vi "Stimulus-Set Level.vi"(0 "Level":T1, 1 "Apply multiplier? (F)":bool, 2 "Name":string, 5 "Waveform in":dbl[](array[numeric]), 11 "error in (no error)":errorcluster) -> (4 "Level out":T1, 6 "Waveform out":dbl[](array[numeric]), 8 "Multiplier":dbl, 10 "Ceiling":dbl, 15 "error out":errorcluster)   [LabVIEW 2020]
uses:
  Controls/Level XCtl/Level Data.ctl
  Controls/Level XCtl/Level Units.ctl
  PXI DAQ VIs/DAQ Engine VIs/PXI Globals.vi
  Utility VIs/Math VIs/dB to Linear (scalar).vi
  Controls/Level XCtl/Level XCtl.xctl
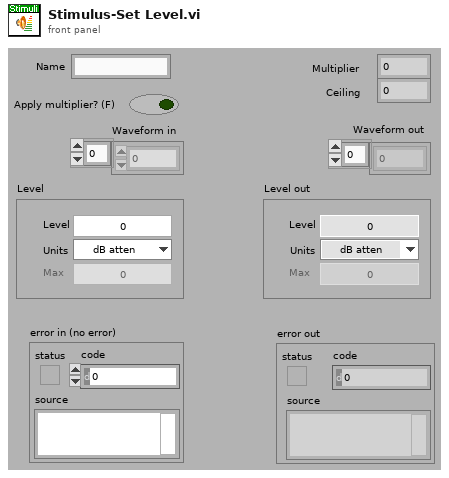
[diagram p1: front panel]
types:
  T1 = typedef "Level XCtl.xctl/Level Data.ctl" = cluster{"Level":dbl, "Units":T2, "Max":dbl, "Multiplier":dbl, "Cal File":path, "Cal":cluster{"Freq (Hz)":dbl[], "Mag (dB SPL)":dbl[], "Phase (deg)":dbl[]}}
  T2 = typedef "Level Units.ctl" = enum16{"dB atten", "dB SPL", "dB re 1 Vrms", "dB V/Hz½", "mW", "dB HL", "Volts", "dB mW"}
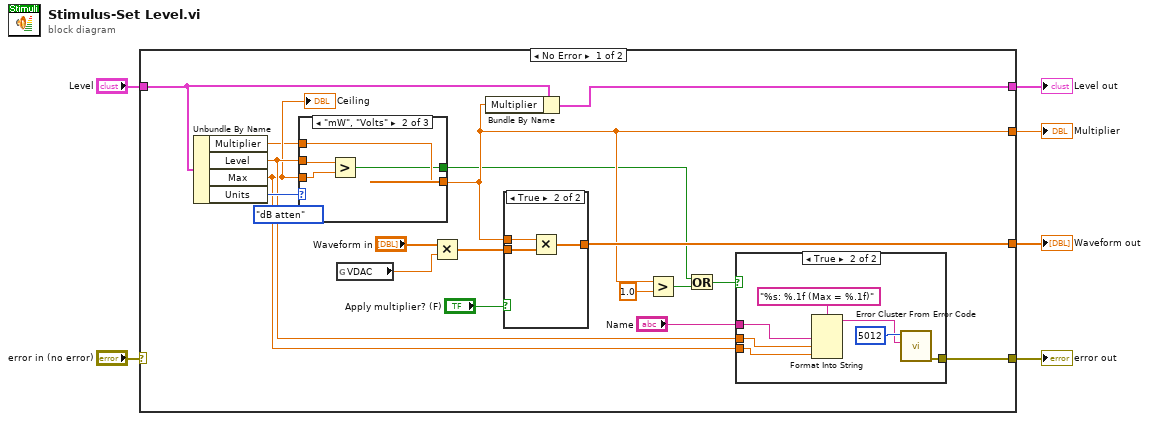
[diagram p0: block diagram]
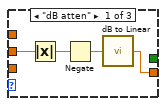
[diagram p4: hidden frame]
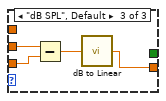
[diagram p5: hidden frame]
diagram:
  n1 = case shown="No Error" "error in (no error)" {
    selector: "error in (no error)" -> [_ w49]
    tunnel: "Level" -> [w24 w48]
    tunnel: [w23 w48] -> w5
    tunnel: [w10 _] -> w4
    tunnel: [w22 _] -> w3
    tunnel: [w15 w49] -> w1
    frame No Error {
      (unwired) Level_Units."dB atten" ("Units")
      n2 = Unbundle By Name(w24) -> ("Multiplier"=w9:dbl, "Level"=w13:dbl, "Max"=w12:dbl, "Units"=w21:T2)
      "Ceiling" <- w12
      n3 = case shown="\"mW\", \"Volts\"" w21 {
        tunnel: w12 -> [_ w41 w47]
        tunnel: w13 -> [w39 w42 w45]
        tunnel: [w36 w43 w44] -> w10
        tunnel: w9 -> [_ w43 _]
        tunnel: [_ w40 _] -> w7
        frame "dB atten" {
          n4 = Absolute Value(x=w39) -> (abs(x)=w38:dbl)
          n5 = Negate(x=w38) -> (-x=w37:dbl)
          n6 = call-poly "dB to Linear.vi"("dB"=w37) -> ("linear"=w36:dbl)
        }
        frame "mW", "Volts" {
          n7 = Greater?(x=w42, y=w41) -> (0:w40:bool)
        }
        frame "dB SPL", Default {
          n8 = Subtract(x=w45, y=w47) -> (x-y=w46:dbl)
          n9 = call-poly "dB to Linear.vi"("dB"=w46) -> ("linear"=w44:dbl)
        }
      }
      n10 = global read "PXI Globals.vi" "VDAC"() -> (w19:dbl)
      n11 = Multiply(x="Waveform in", y=w19) -> (x*y=w17:dbl[])
      n12 = Bundle By Name(cluster=w24, "Multiplier"=w10) -> (w23:T1)
      n13 = case shown="True" "Apply multiplier? (F)" {
        tunnel: w17 -> [w32 w35]
        tunnel: w10 -> [_ w34]
        tunnel: [w32 w33] -> w22
        frame False {
        }
        frame True {
          n14 = Multiply(x=w34, y=w35) -> (x*y=w33:dbl[])
        }
      }
      n15 = Greater?(x=w10, y=1.0) -> (0:w14:bool)
      n16 = Or(x=w7, y=w14) -> (x .or. y?=w8:bool)
      n17 = case shown="True" w8 {
        tunnel: [_ w31] -> w15
        tunnel: w13 -> [_ w26]
        tunnel: w12 -> [_ w28]
        tunnel: "Name" -> [_ w25]
        frame False {
        }
        frame True {
          n18 = Format Into String(format string="%s: %.1f (Max = %.1f)", w25, w26, w28) -> (resulting string=w27:string)  [unwired: 2 in, 1 out]
          n19 = call <vilib>:"Error Cluster From Error Code.vi"("error message (\"\")"=w27, "error code (0)"=5012) -> ("error out"=w31:errorcluster)  [unwired: 7 in]
        }
      }
    }
    frame Error {
    }
  }
  "error out" <- w1
  "Waveform out" <- w3
  "Level out" <- w5
  "Multiplier" <- w4
